vi "deinitialize.vi"(0 "HGF_SVEvent":refnum<class "HGF_SVEvent.lvclass">, 5 "error in (no error)":errorcluster) -> (19 "error out":errorcluster)   [LabVIEW 2012, in "HGF_SV.lvlib" / "HGF_SVEvent.lvclass"]
doc: "This is a dynamic dispatch VI. It can be overwritten by childclasses to release allocated recources."
uses:
  HGF_SVEvent.lvclass
  HGF_BaseClasses/HGF_NetworkEvent/HGF_NetworkEvent.lvclass/HGF_NetworkEvent.lvclass
  HGF_SVEvent.lvclass/HGF_SVEvent.ctl
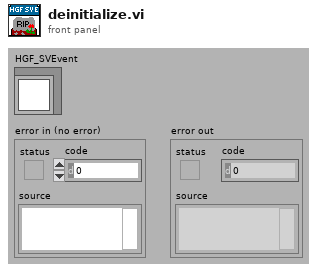
[diagram p1: front panel]
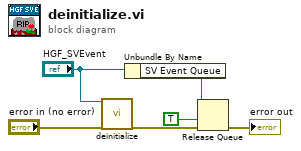
[diagram p0: block diagram]
diagram:
  n1 = call-parent "deinitialize.vi"("HGF_Factory"="HGF_SVEvent", "error in (no error)"="error in (no error)") -> ("error out"=w2:errorcluster)  [unwired: 17 out]
  n2 = Unbundle By Name("HGF_SVEvent") -> ("SV Event Queue"=w4:refnum<queue>)
  n3 = Release Queue(queue=w4, force destroy? (F)=TRUE, error in (no error)=w2) -> (error out=→"error out":errorcluster)  [unwired: 2 out]
